vi "4-Random number on Graph.vi"() -> ()   [LabVIEW 2019]
panel:
  out "Array of a random numbers":dbl[](array[numeric]) format="%#_1g"
  in  "Number of Samples":i32
  out "?":dbl[](graph)
  # "RANDOM NUMBER ON X-Y GRAPH"
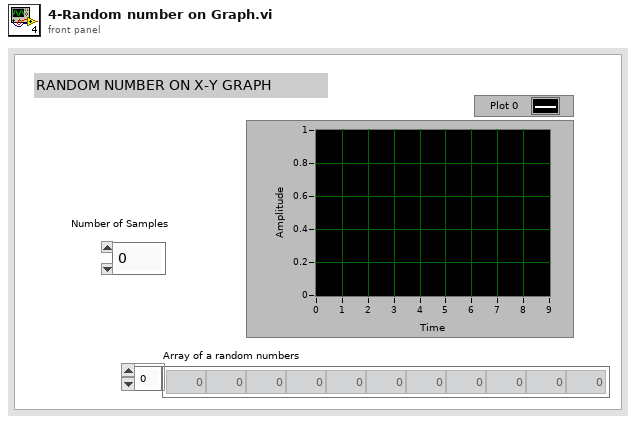
[diagram p1: front panel]
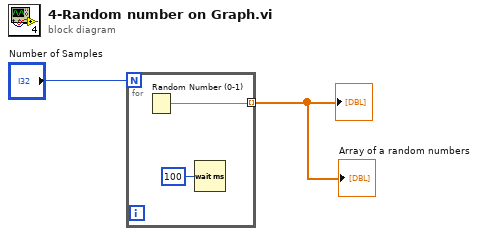
[diagram p0: block diagram]
diagram:
  n1 = for {
    N: "Number of Samples" -> [_]
    tunnel: [w4] -> w1 mode=indexing
    n2 = Random Number (0-1)() -> (number: 0 to 1=w4:dbl)
    n3 = Wait (ms)(milliseconds to wait=u32 100) -> ()  [unwired: 1 out]
  }
  "?" <- w1
  "Array of a random numbers" <- w1
